vi "Read_Write_Text_File.vi"(0 "File_Path_In":path, 5 "Data_In":string, 11 "Error_In":errorcluster, 12 "Mode":T1=enum."Read") -> (4 "File_Path_Out":path, 6 "Data_Out":string, 15 "Error_Out":errorcluster)   [LabVIEW 2021, in "Custom_Sort_Library.lvlib"]
doc: "This VI read or write to the Text file"
uses:
  Custom_Sort_Library.lvlib
  Library_Controls/Mode.ctl
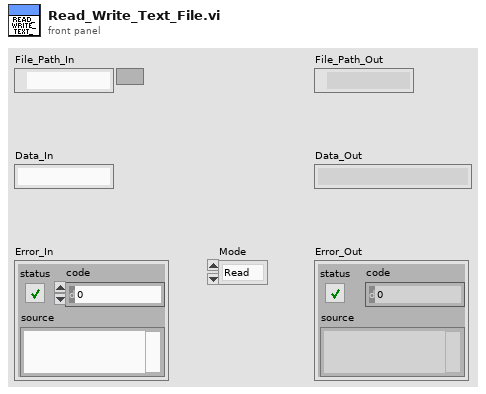
[diagram p1: front panel]
types:
  T1 = typedef "Custom_Sort_Library.lvlib/Mode.ctl" = enum16{"Write", "Read"}
  T2 = enum16{"open", "replace", "create", "open or create", "replace or create", "replace or create with confirmation"}
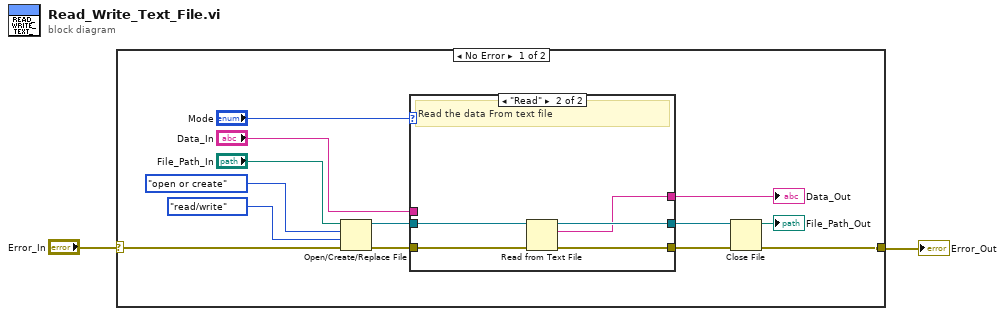
[diagram p0: block diagram]
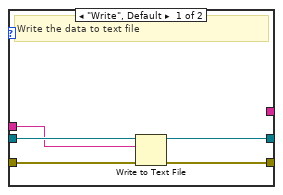
[diagram p2: hidden frame]
diagram:
  n1 = case shown="No Error" "Error_In" {
    selector: "Error_In" -> [w5 w26]
    tunnel: [w4 w26] -> w1
    frame No Error {
      n2 = Open/Create/Replace File(file path (use dialog)="File_Path_In", error in=w5, operation (0:open)=T2."open or create", access (0:read/write)=enum16{"read/write", "read-only", "write-only"}."read/write") -> (refnum out=w12:refnum<file>, error out=w14:errorcluster)  [unwired: 2 in, 1 out]
      n3 = case shown="\"Read\"" "Mode" {
        tunnel: w14 -> [w20 w25]
        tunnel: [w19 w24] -> w13
        tunnel: w12 -> [w18 w22]
        tunnel: "Data_In" -> [w17 _]
        tunnel: [w16 w23] -> w7
        tunnel: [_ w21] -> w6
        frame "Write", Default {
          # "Write the data to text file"
          n4 = Write to Text File(file (use dialog)=w18, text=w17, error in=w20) -> (refnum out=w16:refnum<file>, error out=w19:errorcluster)  [unwired: 1 in, 1 out]
        }
        frame "Read" {
          # "Read the data From text file"
          n5 = Read from Text File(file (use dialog)=w22, error in=w25) -> (refnum out=w23:refnum<file>, text=w21:string, error out=w24:errorcluster)  [unwired: 2 in, 1 out]
        }
      }
      "Data_Out" <- w6
      n6 = Close File(refnum=w7, error in=w13) -> (path=→"File_Path_Out":path, error out=w4:errorcluster)
    }
    frame Error {
    }
  }
  "Error_Out" <- w1
